vi "Wait Event.vi"(8 "error in (no error)":errorcluster, 9 "Timeout mS (-1)":i32=-1, 11 "Promise in":refnum<class "Promise.lvclass">) -> (0 "error out":errorcluster, 2 "Value":refnum<class>, 3 "Promise out":refnum<class "Promise.lvclass">)   [LabVIEW 2020, in "Promises.lvlib" / "Promise.lvclass"]
uses:
  Promise.lvclass
  Promise.lvclass/Promise.ctl
  Error Result/Error Result.lvclass
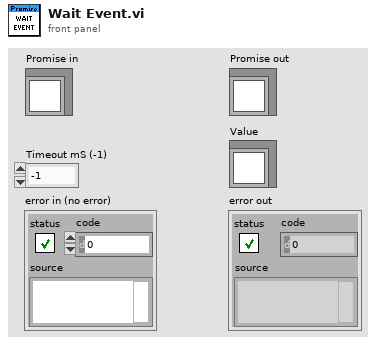
[diagram p1: front panel]
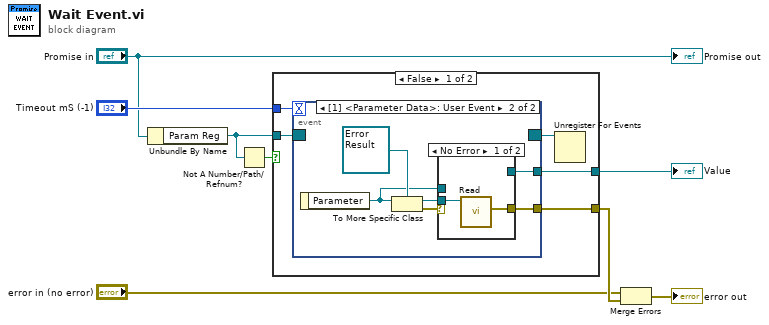
[diagram p0: block diagram]
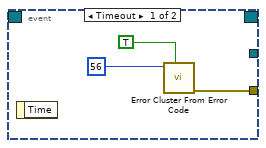
[diagram p2: hidden frame]
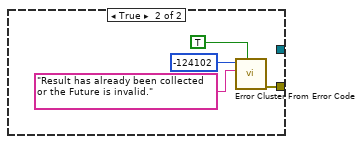
[diagram p4: hidden frame]
diagram:
  n1 = Unbundle By Name("Promise in") -> ("Param Reg"=w8:refnum<event-registration>)
  n2 = Not A Number/Path/Refnum?(number/path/refnum=w8) -> (NaN/Path/Refnum?=w7:bool)
  n3 = case shown="False" w7 {
    tunnel: [w13 _] -> w3
    tunnel: [w12 w29] -> w4
    tunnel: w8 -> [w10 _]
    tunnel: "Timeout mS (-1)" -> [w9 _]
    frame False {
      n4 = event shown="[1] <Parameter Data>: User Event" {
        selector: w10 -> [_ _]
        dyn-events: [_ _] -> w11
        timeout: w9 -> [_ _]
        tunnel: [w14 w22] -> w12
        tunnel: [_ w19] -> w13
        event Timeout {
          n5 = event-data() -> ()  [unwired: 1 in, 1 out]
          n6 = call <vilib>:"Error Cluster From Error Code.vi"("show call chain? (False)"=TRUE, "error code (0)"=56) -> ("error out"=w14:errorcluster)  [unwired: 7 in]
        }
        event User Event {
          n7 = event-data() -> ("Parameter"=w17:refnum<class>)  [unwired: 1 in]
          n8 = To More Specific Class(target class=refnum<class "Error Result.lvclass"> refnum ("Futures:Error Result.lvclass"), reference=w17) -> (specific class reference=w18:refnum<class "Error Result.lvclass">, error out=w21:errorcluster)  [unwired: 1 in]
          n9 = case shown="No Error" w21 {
            tunnel: [w24 _] -> w22
            tunnel: w18 -> [w23 _]
            tunnel: [_ w25] -> w19
            tunnel: w17 -> [_ w25]
            frame No Error {
              n10 = call "Read.vi"("Error Result in"=w23) -> ("Error"=w24:errorcluster)  [unwired: 10 in]
            }
            frame Error {
            }
          }
        }
      }
      n11 = Unregister For Events(event registration refnum=w11) -> ()  [unwired: 1 in, 1 out]
    }
    frame True {
      n12 = call <vilib>:"Error Cluster From Error Code.vi"("show call chain? (False)"=TRUE, "error message (\"\")"="Result has already been collected or the Future is invalid." ("error message (\"\")"), "error code (0)"=-124102) -> ("error out"=w29:errorcluster)  [unwired: 6 in]
    }
  }
  "Value" <- w3
  n13 = Merge Errors("error in (no error)", w4) -> (→"error out":errorcluster)
  "Promise out" <- "Promise in"
